vi "Laser_Power.vi"() -> ()   [LabVIEW 2011]
panel:
  out "?":bool
  in  "Seed Laser Power":i8(knob) min=0 max=100 scale=0.0..100.0
  in  "Laser":bool caption="Seed Laser"
  out "Actual Power Level / [%]":i8(knob) scale=0.0..100.0
  # "Laser Power Settings"
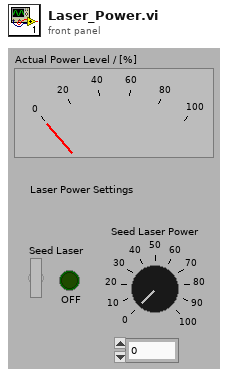
[diagram p1: front panel]
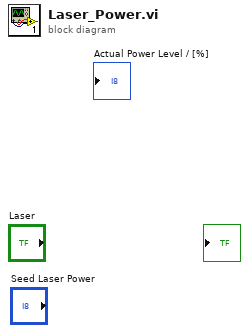
[diagram p0: block diagram]
diagram:
